vi "Riego automático.vi"() -> ()   [LabVIEW 2018]
panel:
  out "B":bool
  out "S":bool
  out "R":bool
  out "D":bool
  out "V":bool
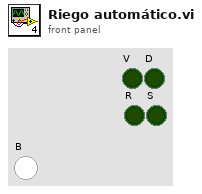
[diagram p1: front panel]
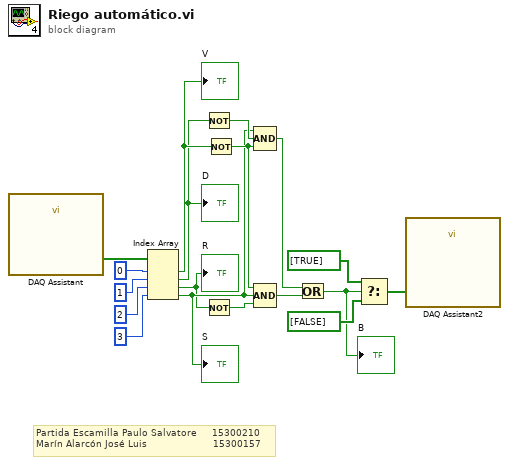
[diagram p0: block diagram]
diagram:
  # "Partida Escamilla Paulo Salvatore     15300210\nMarín Alarcón José Luis                      15300157"
  n1 = call "DAQ Assistant"() -> ("data"=w18:bool[])  [unwired: 17 in, 2 out]
  n2 = Index Array(array=w18, index #1=0 ("index"), index #2=1 ("index"), index #3=2 ("index"), index #4=3 ("index")) -> (element #1=w13:bool, element #2=w9:bool, element #3=w6:bool, element #4=w7:bool)
  "V" <- w13
  "D" <- w9
  "R" <- w6
  "S" <- w7
  n3 = Not(x=w9) -> (.not. x?=w8:bool)
  n4 = Not(x=w6) -> (.not. x?=w5:bool)
  n5 = Not(x=w13) -> (.not. x?=w10:bool)
  n6 = Compound Arithmetic op=AND(w7, w8, w10) -> (w12:bool)
  n7 = Compound Arithmetic op=AND(w10, w7, w5) -> (w11:bool)
  n8 = Or(x=w12, y=w11) -> (x .or. y?=w1:bool)
  "B" <- w1
  n9 = Select(t=bool[] [TRUE] ("data"), s=w1, f=bool[] [FALSE] ("data")) -> (s? t:f=w2:bool[])
  n10 = call "DAQ Assistant2"("data"=w2) -> ()  [unwired: 17 in, 2 out]
